vi "Merge in DB.vi"(0 "DBSet in":refnum<class "DBSet.lvclass">, 5 "SQLite DB Path":path, 11 "error in (no error)":errorcluster {"code" format="Error %.0f"}) -> (4 "DBSet out":refnum<class "DBSet.lvclass">, 15 "error out":errorcluster {"code" format="Error %.0f"})   [LabVIEW 2020, in "DBSet.lvclass"]
uses:
  DBSet.lvclass
  DBSet.lvclass/DBSet.ctl
  <vilib>/drjdpowell/SQLite Library/SQL Statement/SQL Statement.lvclass
  <vilib>/drjdpowell/SQLite Library/Transaction Helpers/Transaction.lvlib
  <vilib>/drjdpowell/SQLite Library/SQL Connection/Connection.lvclass
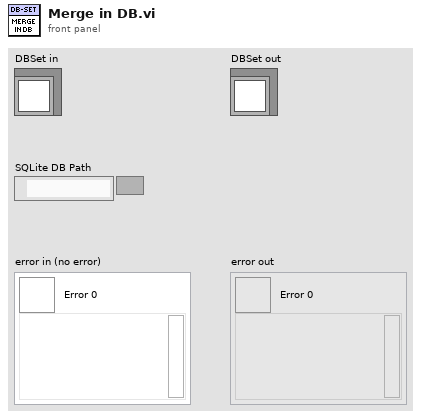
[diagram p1: front panel]
types:
  T1 = typedef "Semaphore RefNum" = refnum<k1>
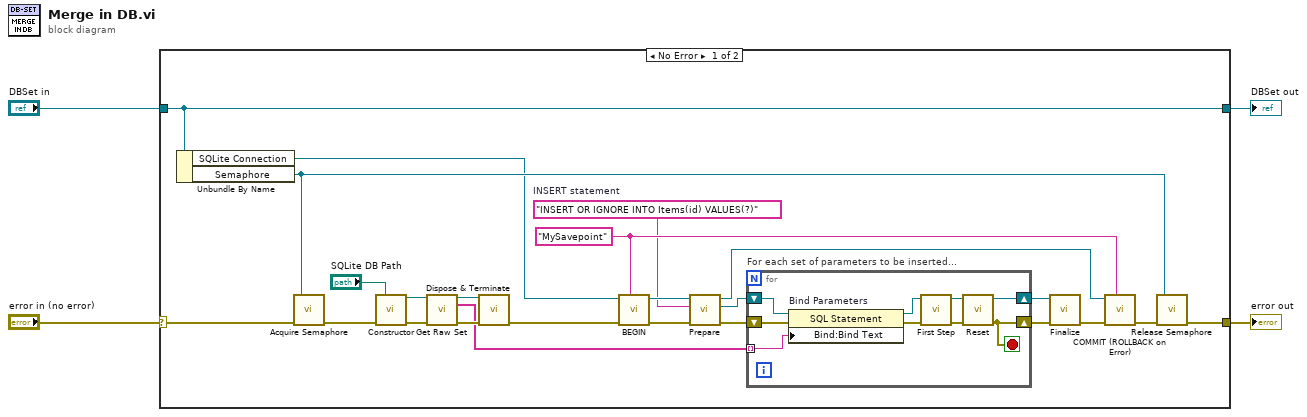
[diagram p0: block diagram]
diagram:
  n1 = case shown="No Error" "error in (no error)" {
    selector: "error in (no error)" -> [w27 w39]
    tunnel: [w26 w39] -> w3
    tunnel: [w28 w38] -> w1
    tunnel: "DBSet in" -> [w28 w38]
    frame No Error {
      w16 = "MySavepoint" ("Savepoint name")
      w11 = "INSERT OR IGNORE INTO Items(id) VALUES(?)"  # INSERT statement
      n2 = Unbundle By Name(w28) -> ("SQLite Connection"=w7:refnum<class "Connection.lvclass">, "Semaphore"=w25:T1)
      n3 = call <vilib>:"Acquire Semaphore.vi"("error in (no error)"=w27, "semaphore"=w25) -> ("error out"=w20:errorcluster)  [unwired: 3 in, 2 out]
      n4 = call "Constructor.vi"("SQLite DB Path"="SQLite DB Path", "error in (no error)"=w20) -> ("DBSet out"=w22:refnum<class "DBSet.lvclass">, "error out"=w24:errorcluster)  [unwired: 12 in]
      n5 = call "Get Raw Set.vi"("DBSet in"=w22, "error in (no error)"=w24) -> ("DBSet out"=w21:refnum<class "DBSet.lvclass">, "Raw Set"=w5:string[], "error out"=w23:errorcluster)  [unwired: 11 in]
      n6 = call-dynamic "Dispose & Terminate.vi"("DBSet in"=w21, "error in (no error)"=w23) -> ("error out"=w6:errorcluster)  [unwired: 12 in, 1 out]
      n7 = call <vilib>:"BEGIN.vi"("Savepoint name"=w16, "error in (no error)"=w6, "SQLite Connection in"=w7) -> ("error out"=w15:errorcluster, "SQLite Connection"=w14:refnum<class "Connection.lvclass">)  [unwired: 7 in]
      n8 = call <vilib>:"Prepare.vi"("error in (no error)"=w15, "SQL"=w11, "SQLite Connection in"=w14) -> ("error out"=w10:errorcluster, "SQL Statement"=w9:refnum<class "SQL Statement.lvclass">, "SQLite Connection"=w17:refnum<class "Connection.lvclass">)  [unwired: 4 in, 2 out]
      n9 = for "For each set of parameters to be inserted..." {
        shift-right: [w31] -> w12
        shift-left: w9 -> [w37]
        shift-right: [w30] -> w13
        shift-left: w10 -> [w34]
        tunnel: w5 -> [w29] mode=indexing
        stop <- w30 stop-if-true
        n10 = property on="Bind Parameters" class="SQL Statement"(reference=w37, error in=w34, "Bind:Bind Text"=w29) -> (reference out=w36:refnum<class "SQL Statement.lvclass">, error out=w35:errorcluster)
        n11 = call <vilib>:"First Step.vi"("error in (no error)"=w35, "SQL Statement in"=w36) -> ("error out"=w33:errorcluster, "SQL Statement"=w32:refnum<class "SQL Statement.lvclass">)  [unwired: 7 in, 1 out]
        n12 = call <vilib>:"Reset.vi"("error in (no error)"=w33, "SQL Statement in"=w32) -> ("error out"=w30:errorcluster, "SQL Statement"=w31:refnum<class "SQL Statement.lvclass">)  [unwired: 8 in]
      }
      n13 = call <vilib>:"Finalize.vi"("error in (no error)"=w13, "SQL Statement in"=w12) -> ("error out"=w18:errorcluster)  [unwired: 9 in]
      n14 = call <vilib>:"COMMIT (ROLLBACK on Error).vi"("Savepoint name"=w16, "error in (no error)"=w18, "SQLite Connection in"=w17) -> ("error out"=w8:errorcluster)  [unwired: 7 in, 1 out]
      n15 = call <vilib>:"Release Semaphore.vi"("error in (no error)"=w8, "semaphore"=w25) -> ("error out"=w26:errorcluster)  [unwired: 4 in, 1 out]
    }
    frame Error {
    }
  }
  "error out" <- w3
  "DBSet out" <- w1
